vi "Attach File to Asset.vi"(8 "error in (no error)":errorcluster, 10 "File ID":string="b2bf3990-d056-4d5e-887b-3075e552995c", 11 "Asset ID":string="2d7e2a0f-e140-47e2-ae68-ae9bd23d949b") -> (0 "error out":errorcluster)   [LabVIEW 2024]
uses:
  <vilib>/Skyline/Configuration/Configuration HTTP_class/NI Skyline Configuration HTTP.lvclass/NI Skyline Configuration HTTP.ctl
  <vilib>/Skyline/Configuration/Configuration HTTP_class/Read Server URL.vi
  <vilib>/Skyline/Configuration/Configuration HTTP_class/Open Configuration HTTP Auto.vi
  <vilib>/httpClient/POSTBuffer.vi
  <vilib>/Skyline/Configuration/Configuration HTTP_class/NI Skyline Configuration HTTP.lvclass
  <vilib>/httpClient/LabVIEWHTTPClient.lvlib
panel:
  out "concatenated string":string
  out "body":string
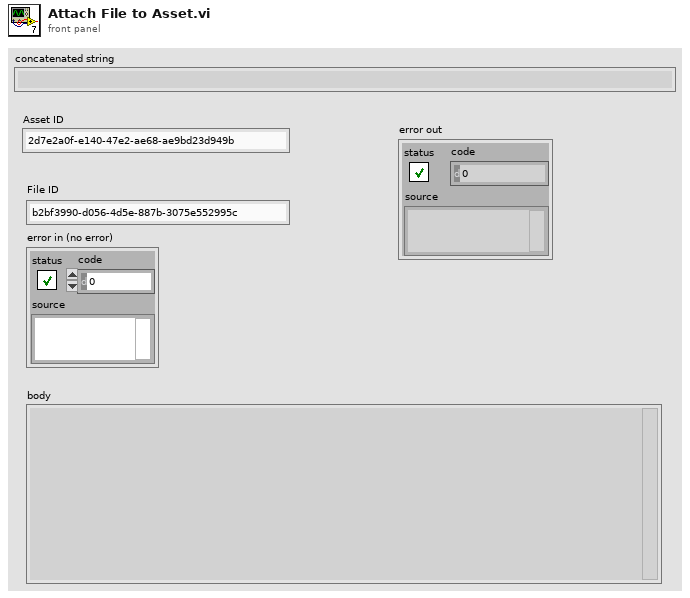
[diagram p1: front panel]
types:
  T1 = typedef "LabVIEWHTTPClient.lvlib/ClientHandle.ctl" = refnum<k1>
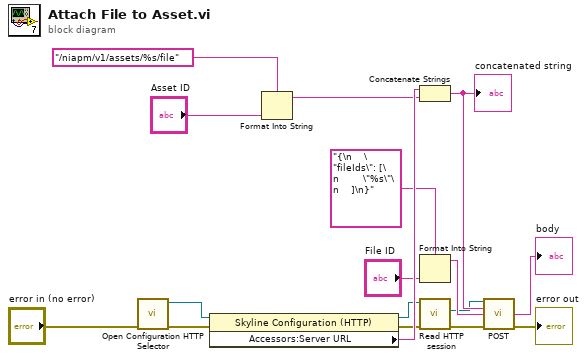
[diagram p0: block diagram]
diagram:
  n1 = call-poly <vilib>:"Open Configuration HTTP Selector.vi"("error in (no error)"="error in (no error)") -> ("error out"=w12:errorcluster, "configuration"=w10:refnum<class "NI Skyline Configuration HTTP.lvclass">)  [unwired: 9 in]
  n2 = property on="Property Node" class="Skyline Configuration (HTTP)"(reference=w10, error in=w12) -> (reference out=w14:refnum<class "NI Skyline Configuration HTTP.lvclass">, error out=w11:errorcluster, "Accessors:Server URL"=w15:string)
  n3 = Format Into String(format string="/niapm/v1/assets/%s/file" ("url"), "Asset ID") -> (resulting string=w4:string)  [unwired: 2 in, 1 out]
  n4 = Concatenate Strings(w15, w4) -> (w16:string)
  "concatenated string" <- w16
  n5 = Format Into String(format string="{\n    \"fileIds\": [\n        \"%s\"\n    ]\n}", "File ID") -> (resulting string=w7:string)  [unwired: 2 in, 1 out]
  n6 = call <vilib>:"Read HTTP session.vi"("error in (no error)"=w11, "HTTP configuration in"=w14) -> ("error out"=w2:errorcluster, "http session"=w3:T1)  [unwired: 7 in, 1 out]
  n7 = call-poly <vilib>:"POST.vi"("client handle"=w3, "url"=w16, "buffer"=w7, "error in (no error)"=w2) -> ("body"=→"body":string, "error out"=→"error out":errorcluster)  [unwired: 8 in, 2 out]
